vi "Character_Clamp.vi"(8 "error in (no error)":errorcluster, 10 "Measurement only":bool, 11 "U8 Character Image In":T1(plugin-control)) -> (0 "error out":errorcluster, 3 "U8 Character Image Out":T1(plugin-control), 4 "Clamp ROI":i32[](array[numeric]))   [LabVIEW 2025]
uses:
  <vilib>/vision/NI_Vision_Development_Module.lvlib
panel:
  out "Row index":i32[](array[numeric])
  out "Column index":i32[](array[numeric])
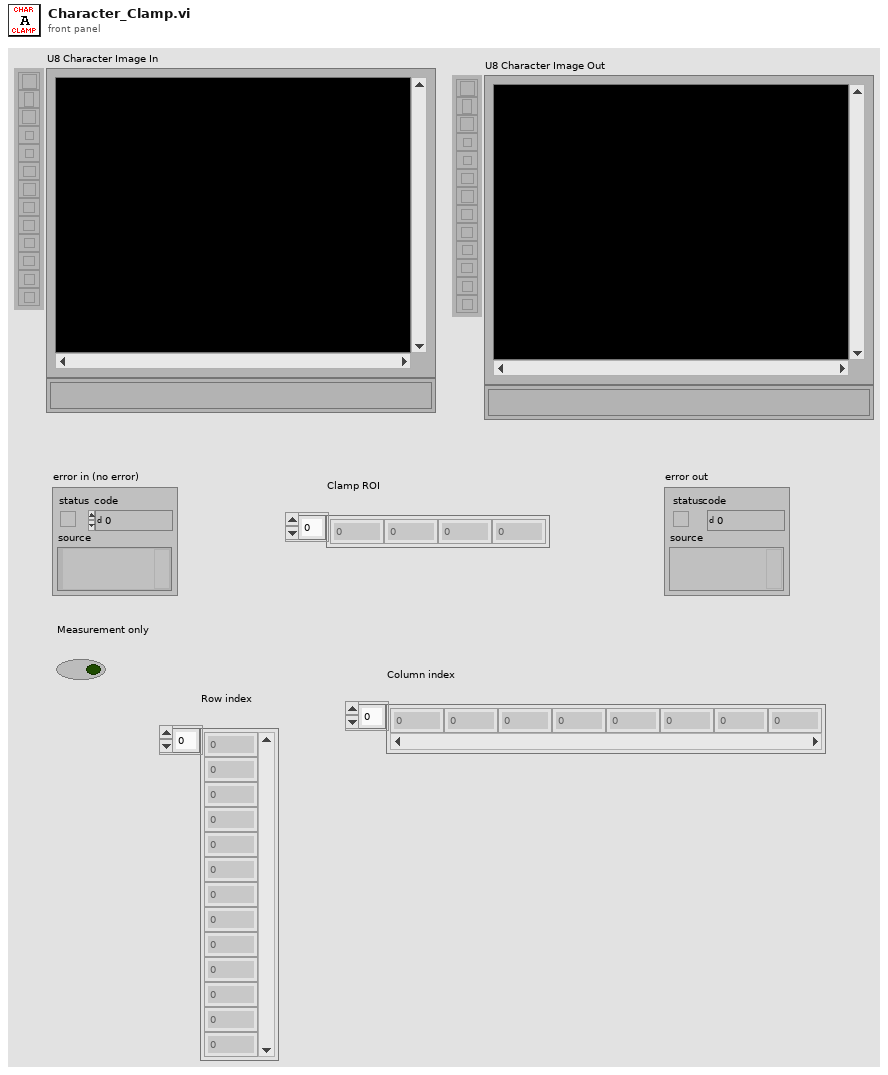
[diagram p1: front panel]
types:
  T1 = typedef "IMAQ Image.ctl" = refnum<image>
  T2 = cluster{"Left":i32, "Top":i32, "Right":i32, "Bottom":i32}
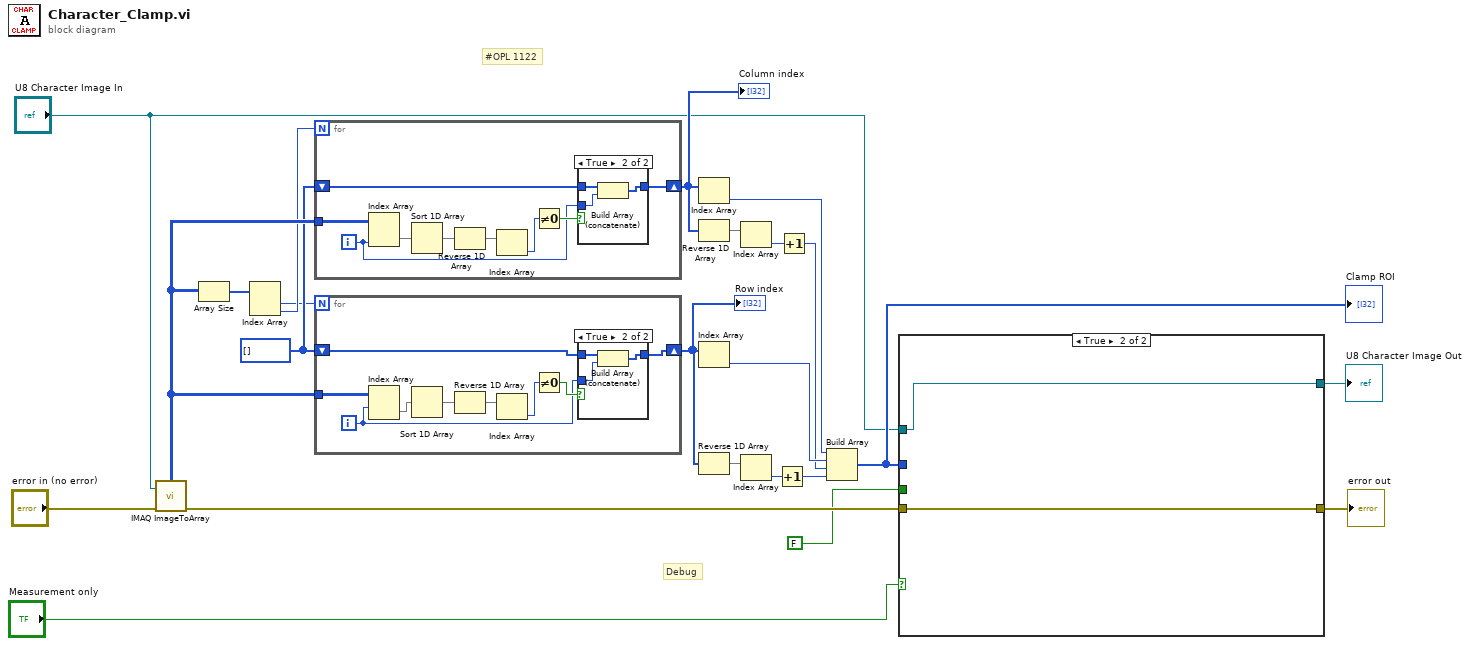
[diagram p0: block diagram]
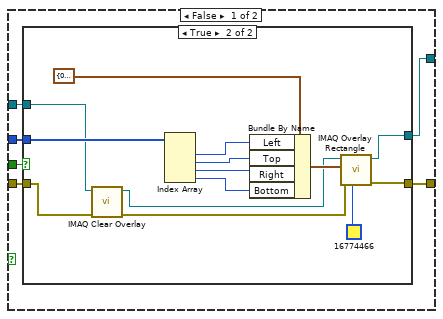
[diagram p2: hidden frame]
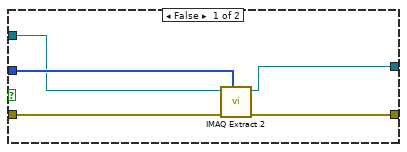
[diagram p3: hidden frame]
diagram:
  w19 = i32[] []
  # "#OPL 1122"
  # "Debug"
  n1 = call "IMAQ ImageToArray"("error in (no error)"="error in (no error)", "Image"="U8 Character Image In") -> ("error out"=w12:errorcluster, "Image Pixels (U8)"=w21:u8[][])  [unwired: 2 in, 3 out]
  n2 = Array Size(array=w21) -> (size(s)=w14:i32[])
  n3 = Index Array(array=w14) -> (element #1=w15:i32, element #2=w20:i32)  [unwired: 2 in]
  n4 = for {
    N: w20 -> [_]
    tunnel: w21 -> [w32]
    shift-right: [w25] -> w17
    shift-left: w19 -> [w26]
    i -> [w24]
    n5 = Index Array(array=w32, index (col)=w24) -> (element=w31:u8[])  [unwired: 1 in]
    n6 = Sort 1D Array(array=w31) -> (sorted array=w30:u8[])
    n7 = Reverse 1D Array(array=w30) -> (reversed array=w29:u8[])
    n8 = Index Array(array=w29) -> (element=w28:u8)  [unwired: 1 in]
    n9 = Not Equal To 0?(x=w28) -> (x != 0?=w27:bool)
    n10 = case shown="True" w27 {
      tunnel: w24 -> [_ w35]
      tunnel: w26 -> [w33 w36]
      tunnel: [w33 w34] -> w25
      frame False {
      }
      frame True {
        n11 = Build Array (concatenate)(w36, w35) -> (w34:i32[])
      }
    }
  }
  "Column index" <- w17
  n12 = for {
    N: w15 -> [_]
    tunnel: w21 -> [w45]
    shift-right: [w37] -> w6
    shift-left: w19 -> [w38]
    i -> [w39]
    n13 = Index Array(array=w45, index (row)=w39) -> (element=w44:u8[])  [unwired: 1 in]
    n14 = Sort 1D Array(array=w44) -> (sorted array=w43:u8[])
    n15 = Reverse 1D Array(array=w43) -> (reversed array=w42:u8[])
    n16 = Index Array(array=w42) -> (element=w41:u8)  [unwired: 1 in]
    n17 = Not Equal To 0?(x=w41) -> (x != 0?=w40:bool)
    n18 = case shown="True" w40 {
      tunnel: w39 -> [_ w48]
      tunnel: w38 -> [w46 w49]
      tunnel: [w46 w47] -> w37
      frame False {
      }
      frame True {
        n19 = Build Array (concatenate)(w49, w48) -> (w47:i32[])
      }
    }
  }
  "Row index" <- w6
  n20 = Index Array(array=w17) -> (element=w7:i32)  [unwired: 1 in]
  n21 = Reverse 1D Array(array=w17) -> (reversed array=w18:i32[])
  n22 = Index Array(array=w6) -> (element=w8:i32)  [unwired: 1 in]
  n23 = Reverse 1D Array(array=w6) -> (reversed array=w16:i32[])
  n24 = Index Array(array=w18) -> (element=w5:i32)  [unwired: 1 in]
  n25 = Index Array(array=w16) -> (element=w3:i32)  [unwired: 1 in]
  n26 = Increment(x=w3) -> (x+1=w2:i32)
  n27 = Increment(x=w5) -> (x+1=w4:i32)
  n28 = Build Array(w7, w8, w4, w2) -> (w22:i32[])
  "Clamp ROI" <- w22
  n29 = case shown="True" "Measurement only" {
    tunnel: [w55 w76] -> w23
    tunnel: w22 -> [w54 _]
    tunnel: "U8 Character Image In" -> [w53 w76]
    tunnel: w12 -> [w52 w75]
    tunnel: [w51 w75] -> w10
    tunnel: FALSE -> [w50 _]
    frame False {
      n30 = case shown="True" w50 {
        tunnel: [w60 w66] -> w55
        tunnel: w54 -> [w59 w73]
        tunnel: w53 -> [w58 w62]
        tunnel: w52 -> [w57 w64]
        tunnel: [w56 w67] -> w51
        frame False {
          n31 = call "IMAQ Extract 2"("Optional Rectangle"=w59, "error in (no error)"=w57, "Image Src"=w58) -> ("error out"=w56:errorcluster, "Image Dst Out"=w60:T1)  [unwired: 7 in]
        }
        frame True {
          n32 = call "IMAQ Clear Overlay"("error in (no error)"=w64, "Image"=w62) -> ("error out"=w63:errorcluster, "Image Out"=w61:T1)  [unwired: 8 in]
          n33 = Index Array(array=w73) -> (element #1=w72:i32, element #2=w71:i32, element #3=w70:i32, element #4=w69:i32)  [unwired: 4 in]
          n34 = Bundle By Name(cluster=T2 {"Left"=0, "Top"=0, "Right"=0, "Bottom"=0} ("Rectangle"), "Left"=w72, "Top"=w71, "Right"=w70, "Bottom"=w69) -> (w68:T2)
          n35 = call "IMAQ Overlay Rectangle"("Color"=u32 16774466, "error in (no error)"=w63, "Rectangle"=w68, "Image"=w61) -> ("error out"=w67:errorcluster, "Image Out"=w66:T1)  [unwired: 6 in]
        }
      }
    }
    frame True {
    }
  }
  "U8 Character Image Out" <- w23
  "error out" <- w10
